vi "FIR Filter by N Specs for N Chan (CDB).vi"(4 "optional FIR filter specifications":T2(array[cluster]) {"SB Gain" format="%0.2f"; "PB Gain" format="%0.2f"}, 6 "FIR filter specifications":T3(array[cluster]) {"Lower SB" format="%0.2p"; "Upper SB" format="%0.2p"; "Lower PB" format="%0.2p"; "Upper PB" format="%0.2p"}, 7 "reset filters":bool, 8 "error in (no error)":errorcluster, 11 "signal(s) in":waveform(cdb)[](array[waveform])) -> (0 "error out":errorcluster, 2 "filter information":T1(array[cluster]) {"phase H(w)"."df" format="%0.2f"; "phase H(w)"."f0" format="%0.2f"; "phase H(w)"."Phase H(w)" format="%0.2f"; "magnitude H(w)"."df" format="%0.2f"; "magnitude H(w)"."f0" format="%0.2f"; "magnitude H(w)"."Mag H(w)" format="%0.2f"}, 3 "signal(s) out":waveform(cdb)[](array[waveform]))   [LabVIEW 2020, in "NI_MAPro.lvlib"]
doc: "Filters signals in either single or multiple waveforms. If you are filtering multiple waveforms, the VI maintains separate filter states for each waveform. The data types you wire to the <B>signal in</B> and <B>FIR filter specifications</B> inputs determine the polymorphic instance to use."
uses:
  NI_MAPro.lvlib
  NI_MABase.lvlib
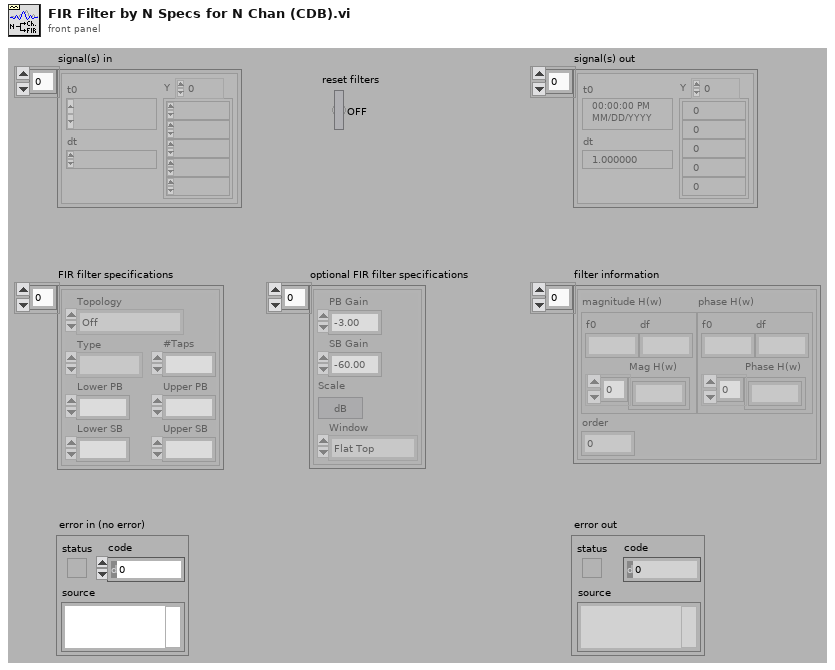
[diagram p1: front panel]
types:
  T1 = cluster{"magnitude H(w)":cluster{"f0":dbl, "df":dbl, "Mag H(w)":dbl[]}, "phase H(w)":cluster{"f0":dbl, "df":dbl, "Phase H(w)":dbl[]}, "order":i32}[]
  T2 = cluster{"PB Gain":dbl, "SB Gain":dbl, "Scale":bool, "Window":enum16{"None", "Hanning", "Hamming", "Triangular", "Blackman", "Exact Blackman", "Blackman-Harris", "Kaiser-Bessel", "Flat Top"}}[]
  T3 = cluster{"Topology":enum16{"Off", "FIR by Specification", "Equi-ripple FIR", "Windowed FIR"}, "Type":enum16{"Lowpass", "Highpass", "Bandpass", "Bandstop"}, "#Taps":i32, "Lower PB":dbl, "Upper PB":dbl, "Lower SB":dbl, "Upper SB":dbl}[]
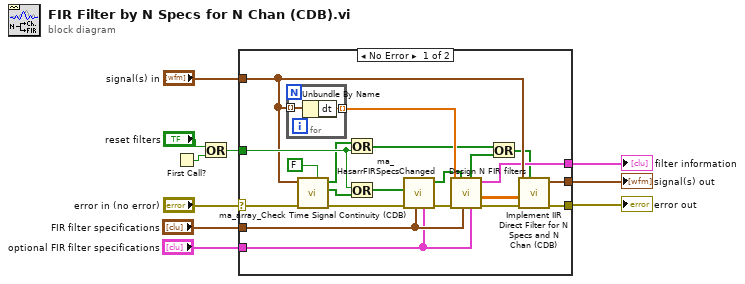
[diagram p0: block diagram]
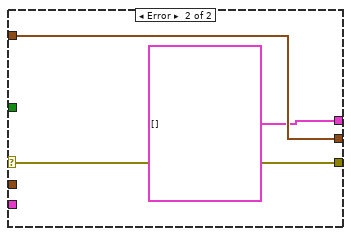
[diagram p2: hidden frame]
diagram:
  n1 = First Call?() -> (First Call?: T/F=w4:bool)
  n2 = Or(x="reset filters", y=w4) -> (x .or. y?=w2:bool)
  n3 = case shown="No Error" "error in (no error)" {
    selector: "error in (no error)" -> [w25 w35]
    tunnel: "FIR filter specifications" -> [w30 _]
    tunnel: [w31 w35] -> w10
    tunnel: w2 -> [w28 _]
    tunnel: [w27 w36] -> w8
    tunnel: "optional FIR filter specifications" -> [w29 _]
    tunnel: "signal(s) in" -> [w26 w36]
    tunnel: [w24 T1 [] ("arrFilterInfo")] -> w1
    frame No Error {
      n4 = for {
        tunnel: w26 -> [w33] mode=indexing
        tunnel: [w32] -> w21 mode=indexing
        n5 = Unbundle By Name(w33) -> ("dt"=w32:dbl)
      }
      n6 = call "ma_array_Check Time Signal Continuity (CDB).vi"("Ignore input time stamp"=FALSE, "error in (no error)"=w25, "waveforms"=w26) -> ("error out"=w17:errorcluster, "dt changed"=w14:bool[], "t0 changed"=w13:bool[])  [unwired: 5 in, 1 out]
      n7 = Or(x=w13, y=w28) -> (x .or. y?=w12:bool[])
      n8 = Or(x=w28, y=w14) -> (x .or. y?=w15:bool[])
      n9 = call "ma_HasarrFIRSpecsChanged.vi"("optional IIR filter specifications"=w29, "IIR filter specs"=w30, "error in (no error)"=w17, "redesign filter"=w15) -> ("error out"=w18:errorcluster, "valsDifferent?"=w16:bool[])  [unwired: 6 in]
      n10 = call "Design N FIR filters.vi"("arrOptionalFilterSpecs"=w29, "arrFilterSpecs"=w30, "redesign filters"=w16, "error in"=w18, "arrdt"=w21) -> ("error out"=w22:errorcluster, "arrForward Coefficients"=w23:dbl[][], "arrFilterInfo"=w24:T1, "reset filter states"=w19:bool[])  [unwired: 3 in]
      n11 = Or(x=w12, y=w19) -> (x .or. y?=w20:bool[])
      n12 = call "Implement IIR Direct Filter for N Specs and N Chan (CDB).vi"("reset Filters"=w20, "error in (no error)"=w22, "Forward Coefficients"=w23, "arrWaveforms In"=w26) -> ("error out"=w31:errorcluster, "arrWaveforms Out"=w27:waveform(cdb)[])  [unwired: 6 in]
    }
    frame Error {
    }
  }
  "error out" <- w10
  "signal(s) out" <- w8
  "filter information" <- w1
